vi "passTestMaintainsBallPossesion.vi"(8 "Kicker robot":T2, 9 "IA state":T3, 10 "Receveing robot":T2) -> (4 "Result":T1)   [LabVIEW 2017]
uses:
  <extravilib>/ChannelInstances/Lossy Stream-dbl/)Channel.ctl
  <extravilib>/ChannelInstances/Lossy Stream-t'AI Input.ctl'/)Channel.ctl
  Core/AI Input.ctl
  Core/AI Robot.ctl
  Intel/Functions Enum.ctl
  Intel/AttackerStates.ctl
  Core/AI Ball.ctl
  Core/Field Size.ctl
  Core/AI Judge.ctl
  Intel/Command Enum.ctl
  Util/Events/Events.ctl
  <extravilib>/ChannelInstances/Lossy Stream-t'passTestStates.ctl'/)Channel.ctl
  passTestStates.ctl
  <extravilib>/ChannelInstances/Lossy Stream-dbl/Read With Abort.vi
  <extravilib>/ChannelInstances/Lossy Stream-t'AI Input.ctl'/Read With Abort.vi
  <extravilib>/ChannelInstances/Lossy Stream-t'passTestStates.ctl'/Write With Abort.vi
  <extravilib>/ChannelInstances/Lossy Stream-dbl/EndpointRead.vi
  <extravilib>/ChannelInstances/Lossy Stream-t'AI Input.ctl'/EndpointRead.vi
  <extravilib>/ChannelInstances/Lossy Stream-t'passTestStates.ctl'/Endpoint.vi
  <extravilib>/ChannelInstances/Lossy Stream-dbl/)Channel.vi
  <resource>/ChannelSupport/_ChannelSupport/WaitIfNeeded.vi
  <extravilib>/ChannelInstances/Lossy Stream-t'AI Input.ctl'/)Channel.vi
  <extravilib>/ChannelInstances/Lossy Stream-t'passTestStates.ctl'/)Channel.vi
  <extravilib>/ChannelInstances/Lossy Stream-t'passTestStates.ctl'.lvlib
  <extravilib>/ChannelInstances/Lossy Stream-t'AI Input.ctl'.lvlib
  <extravilib>/ChannelInstances/Lossy Stream-dbl.lvlib
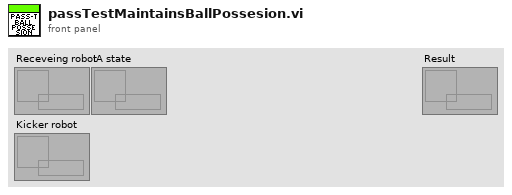
[diagram p1: front panel]
types:
  T1 = typedef "Lossy Stream-t'passTestStates.ctl'.lvlib/)Channel.ctl" = refnum<queue>
  T2 = typedef "Lossy Stream-dbl.lvlib/)Channel.ctl" = refnum<queue>
  T3 = typedef "Lossy Stream-t'AI Input.ctl'.lvlib/)Channel.ctl" = refnum<queue>
  T4 = typedef "passTestStates.ctl" = enum16{"Pass on the way", "Ball stops", "Pass intercepted", "Ball out of the field", "Ball missed robot", "Need more force to pass", "Too much force", "Correct pass", "Keep ball possesion", "Robot kicked the ball", "Waiting Kick", "Invalid: same robot", "Invalid: kicker ID 999", "Invalid: Receiver ID 999", "Invalid"}
  T5 = typedef "AI Input.ctl" = cluster{"our_robots":T6[], "enemy_robots":T6[], "balls":T9[], "geometry":T10, "IA Judge":T11, "Received Timestamp":timestamp, "Events":T13}
  T6 = typedef "AI Robot.ctl" = cluster{"id":u32, "function":T7, "x":dbl, "y":dbl, "orientation":dbl, "v_tangent":dbl, "v_normal":dbl, "v_ang":dbl, "kick_x":dbl, "kick_z":dbl, "dribble":bool, "Timestamp":timestamp, "dest_x":dbl, "dest_y":dbl, "dest_orientation":dbl, "estimatives":cluster{"est_v_tangent":dbl, "est_v_normal":dbl, "est_vx":dbl, "est_vy":dbl, "Pos Robot Est":dbl[]}, "dest_x_kick":dbl, "dest_y_kick":dbl, "Gap Coord":dbl[], "States":T8}
  T7 = typedef "Functions Enum.ctl" = enum16{"Attacker", "Goalie", "Defender", "Striker", "Goto 0", "Dummy", "Kicker", "ZigZag"}
  T8 = typedef "AttackerStates.ctl" = enum16{"Pass", "GoToTangent", "BallGetting", "GoToKick", ""}
  T9 = typedef "AI Ball.ctl" = cluster{"x":dbl, "y":dbl, "timestamp":timestamp, "Vel_x":dbl, "Vel_y":dbl, "Pos Bola Est":dbl[]}
  T10 = typedef "Field Size.ctl" = cluster{"line_width":u32, "field_length":u32, "field_width":u32, "boundary_width":u32, "referee_width":u32, "goal_width":u32, "goal_depth":u32, "goal_wall_width":u32, "center_circle_radius":u32, "defense_radius":u32, "defense_stretch":u32, "free_kick_from_defense_dist":u32, "penalty_spot_from_field_line_dist":u32, "penalty_line_from_spot_dist":u32}
  T11 = typedef "AI Judge.ctl" = cluster{"stage":string, "command":string, "our_goalie_id":dbl, "enemy_goalie_id":dbl, "command enum":T12, "Time":enum16{"Azul", "Amarelo"}}
  T12 = typedef "Command Enum.ctl" = enum16{"Halt", "Stop", "Force Start", "PKA Normal Start", "Prepare Kickoff Ally", "PKE Normal Start", "Prepare Kickoff Enemy", "Prepare Penalty Ally", "PPA Normal Start", "Prepare Penalty Enemy", "PPE Normal Start", "Direct Free Enemy", "Direct Free Ally", "Indirect Free Enemy", "Indirect Free Ally", "Timeout Enemy", "Timeout Ally", "Goal Enemy", "Goal Ally", "Ball Placement Enemy", "Ball Placement Ally", "Normal Half Time", "Extra Time Break", "Extra Half Time", "None", "Post Game"}
  T13 = typedef "Events.ctl" = cluster{"Touch":bool, "Ball out":bool, "id touch":dbl, "Ball out of \nVision":bool, "Ball inside \nGoalie area":bool, "Robot not responding":bool, "Robots responding status":dbl[], "Enemy Ball \nPossession":bool, "Pass State":bool, "id end of pass":dbl, "Kick":bool, "Id ini Possession":dbl, "Ball Possesion":bool, "Id Possesion":dbl}
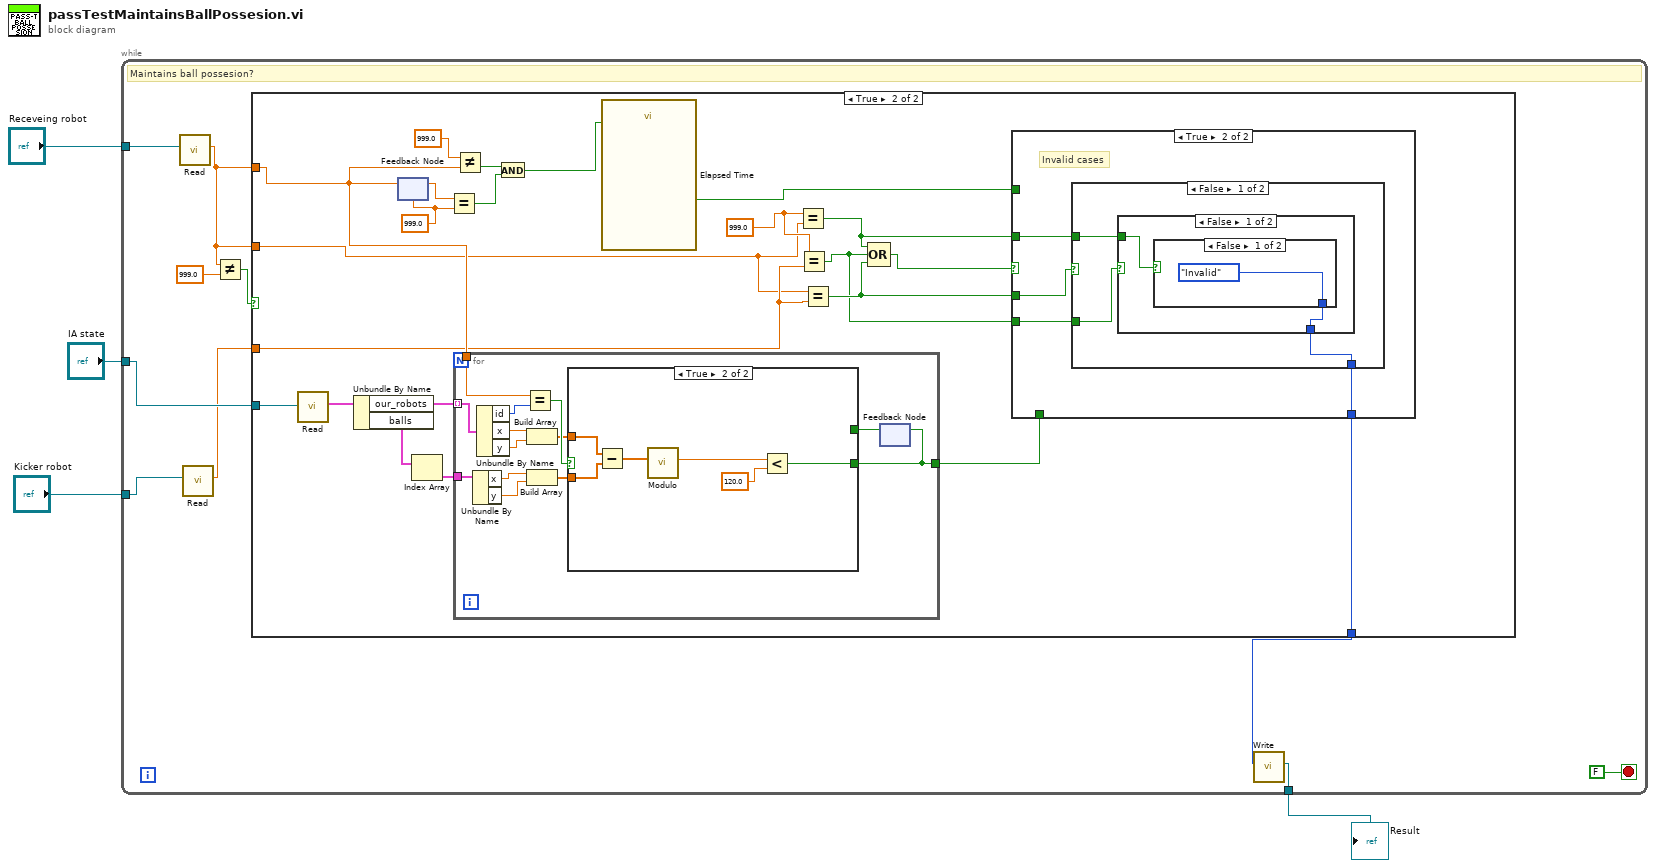
[diagram p0: block diagram]
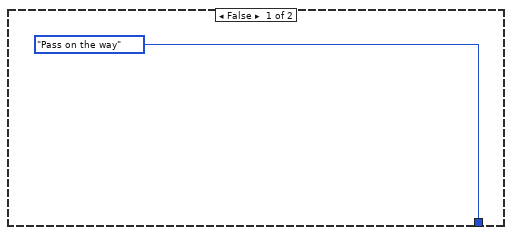
[diagram p2: hidden frame]
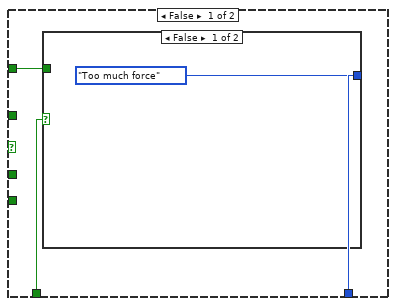
[diagram p3: hidden frame]
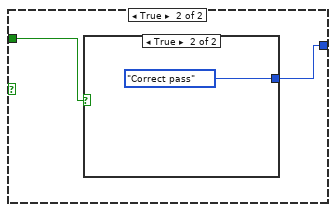
[diagram p4: hidden frame]
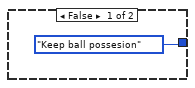
[diagram p5: hidden frame]
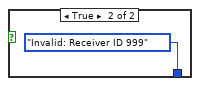
[diagram p6: hidden frame]
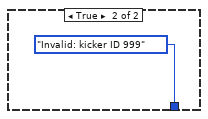
[diagram p7: hidden frame]
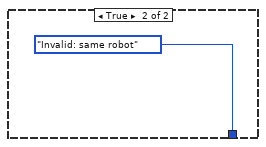
[diagram p8: hidden frame]
diagram:
  n1 = while {
    tunnel: "Receveing robot" -> [w11]
    tunnel: [w12] -> w1
    tunnel: "IA state" -> [w8]
    tunnel: "Kicker robot" -> [w7]
    stop <- FALSE stop-if-true
    # "Maintains ball possesion?"
    n2 = call <extravilib>:"Read.vi"("channel"=w11) -> ("element"=w5:dbl)  [unwired: 5 in, 5 out]
    n3 = call <extravilib>:"Read.vi"("channel"=w7) -> ("element"=w6:dbl)  [unwired: 5 in, 5 out]
    n4 = Not Equal?(x=w5, y=999.0) -> (x != y?=w9:bool)
    n5 = case shown="True" w9 {
      tunnel: w8 -> [_ w37]
      tunnel: [passTestStates."Pass on the way" w29] -> w13
      tunnel: w5 -> [_ w26]
      tunnel: w6 -> [_ w21]
      tunnel: w5 -> [_ w20]
      frame False {
      }
      frame True {
        w22 = 999.0 ("x")
        w36 = 999.0 ("element")
        n6 = call <extravilib>:"Read.vi"("channel"=w37) -> ("element"=w28:T5)  [unwired: 5 in, 5 out]
        n7 = Unbundle By Name(w28) -> ("our_robots"=w27:T6[], "balls"=w25:T9[])
        n8 = feedback #1(w36) -> (w35:dbl)
        n9 = feedback-in #1(w26) -> ()
        n10 = Index Array(array=w25) -> (element=w24:T9)  [unwired: 1 in]
        n11 = Equal?(x=w35, y=w36) -> (x = y?=w34:bool)
        n12 = for {
          tunnel: w27 -> [w71] mode=indexing
          tunnel: w26 -> [w69]
          tunnel: w24 -> [w65]
          tunnel: [w60] -> w23
          n13 = Unbundle By Name(w65) -> ("x"=w64:dbl, "y"=w63:dbl)
          n14 = Unbundle By Name(w71) -> ("id"=w70:u32, "x"=w67:dbl, "y"=w66:dbl)
          n15 = Equal?(x=w69, y=w70) -> (x = y?=w68:bool)
          n16 = Build Array(w67, w66) -> (w62:dbl[])
          n17 = Build Array(w64, w63) -> (w61:dbl[])
          n18 = feedback #2() -> (w59:bool)  [unwired: 1 in]
          n19 = case shown="True" w68 {
            tunnel: w62 -> [_ w78]
            tunnel: w61 -> [_ w77]
            tunnel: [w72 w73] -> w60
            tunnel: w59 -> [w72 _]
            frame False {
            }
            frame True {
              n20 = Subtract(x=w78, y=w77) -> (x-y=w76:dbl[])
              n21 = call "Modulo.vi"("2D vector"=w76) -> ("Modulo"=w75:dbl)  [unwired: 10 in]
              n22 = Less?(x=w75, y=120.0) -> (x < y?=w73:bool)
            }
          }
          n23 = feedback-in #2(w60) -> ()
        }
        n24 = Not Equal?(x=999.0 ("element"), y=w26) -> (x != y?=w33:bool)
        n25 = And(x=w33, y=w34) -> (x .and. y?=w31:bool)
        n26 = call "Elapsed Time"("Reset"=w31) -> ("Time has Elapsed"=w30:bool)  [unwired: 11 in, 7 out]
        n27 = Equal?(x=w22, y=w20) -> (x = y?=w16:bool)
        n28 = Equal?(x=w22, y=w21) -> (x = y?=w17:bool)
        n29 = Equal?(x=w20, y=w21) -> (x = y?=w18:bool)
        n30 = Compound Arithmetic op=OR(w16, w17, w18) -> (w19:bool)
        n31 = case shown="True" w19 {
          tunnel: w30 -> [w40 _]
          tunnel: [w39 w49] -> w29
          tunnel: w23 -> [w38 _]
          tunnel: w18 -> [_ w48]
          tunnel: w17 -> [_ w47]
          tunnel: w16 -> [_ w46]
          frame False {
            n32 = case shown="False" w38 {
              tunnel: [passTestStates."Too much force" w43] -> w39
              tunnel: w40 -> [_ w42]
              frame False {
              }
              frame True {
                n33 = case shown="True" w42 {
                  tunnel: [passTestStates."Keep ball possesion" passTestStates."Correct pass"] -> w43
                  frame False {
                  }
                  frame True {
                  }
                }
              }
            }
          }
          frame True {
            # "Invalid cases"
            n34 = case shown="False" w48 {
              tunnel: [w52 passTestStates."Invalid: same robot"] -> w49
              tunnel: w47 -> [w51 _]
              tunnel: w46 -> [w50 _]
              frame False {
                n35 = case shown="False" w51 {
                  tunnel: [w54 passTestStates."Invalid: kicker ID 999"] -> w52
                  tunnel: w50 -> [w53 _]
                  frame False {
                    n36 = case shown="False" w53 {
                      tunnel: [passTestStates."Invalid" passTestStates."Invalid: Receiver ID 999"] -> w54
                      frame False {
                      }
                      frame True {
                      }
                    }
                  }
                  frame True {
                  }
                }
              }
              frame True {
              }
            }
          }
        }
      }
    }
    n37 = call <extravilib>:"Write.vi"("element"=w13) -> ("channel"=w12:T1)  [unwired: 8 in, 2 out]
  }
  "Result" <- w1
